vi "TAGs_AURAwheel.vi"(0 "Nº Ejes":i32[](array[numeric]), 1 "TAGs":string[](array[string]), 2 "Ejes_convoy":i32, 3 "it-LR6":i32, 4 "TAGs LR6":string[](array[string]), 5 "it-read-LR6":i32[](array[numeric]), 8 "Plataformas?":bool) -> (7 "TAGS_AURA":string[][](array[string]))   [LabVIEW 2015]
panel:
  out "x > y?":bool
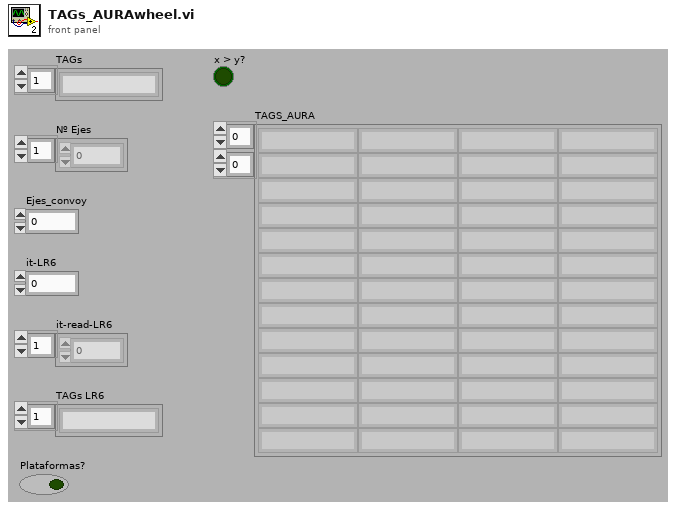
[diagram p1: front panel]
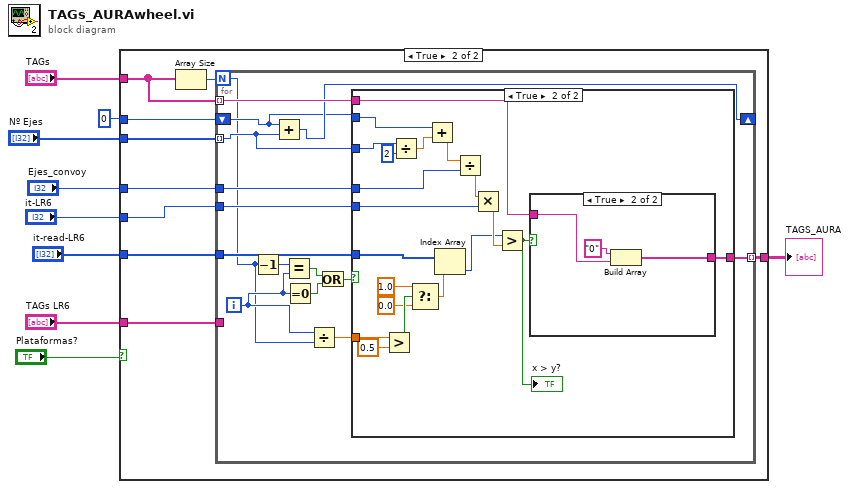
[diagram p0: block diagram]
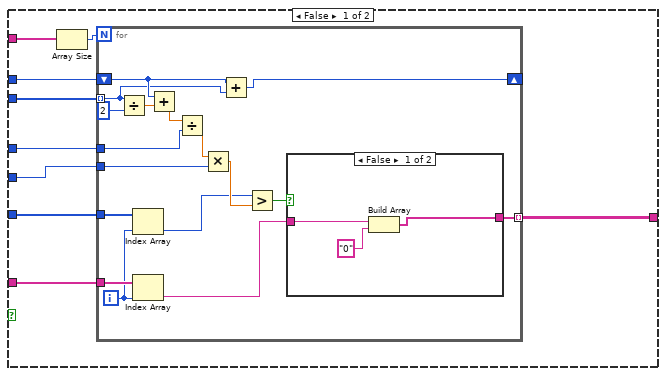
[diagram p2: hidden frame]
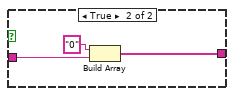
[diagram p3: hidden frame]
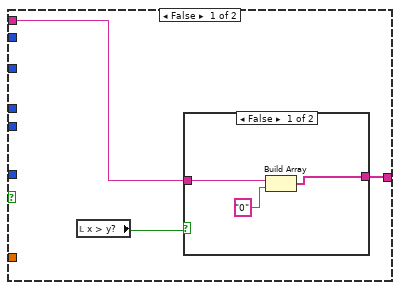
[diagram p4: hidden frame]
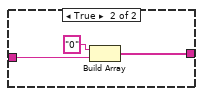
[diagram p5: hidden frame]
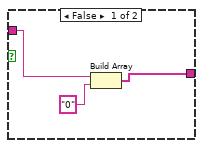
[diagram p6: hidden frame]
diagram:
  n1 = case shown="True" "Plataformas?" {
    tunnel: "TAGs LR6" -> [w17 w45]
    tunnel: "it-LR6" -> [w13 w47]
    tunnel: "it-read-LR6" -> [w16 w46]
    tunnel: "Nº Ejes" -> [w15 w49]
    tunnel: "Ejes_convoy" -> [w14 w48]
    tunnel: "TAGs" -> [w12 w43]
    tunnel: [w11 w44] -> w8
    tunnel: 0 -> [w10 w42]
    frame False {
      n2 = Array Size(array=w12) -> (size(s)=w18:i32)
      n3 = for {
        N: w18 -> [_]
        tunnel: w17 -> [w35]
        tunnel: w16 -> [w34]
        tunnel: w15 -> [w20] mode=indexing
        tunnel: w14 -> [w31]
        tunnel: w13 -> [w29]
        tunnel: [w24] -> w11 mode=indexing
        shift-right: [w19] -> _
        shift-left: w10 -> [w21]
        i -> [w33]
        n4 = Divide(x=w20, y=2) -> (x/y=w23:dbl)
        n5 = Index Array(array=w34, index=w33) -> (element=w27:i32)
        n6 = Index Array(array=w35, index=w33) -> (element=w25:string)
        n7 = Add(x=w21, y=w23) -> (x+y=w22:dbl)
        n8 = Divide(x=w22, y=w31) -> (x/y=w30:dbl)
        n9 = Multiply(x=w30, y=w29) -> (x*y=w28:dbl)
        n10 = Add(x=w21, y=w20) -> (x+y=w19:i32)
        n11 = Greater?(x=w27, y=w28) -> (0:w26:bool)
        n12 = case shown="False" w26 {
          tunnel: w25 -> [w37 w41]
          tunnel: [w36 w39] -> w24
          frame False {
            n13 = Build Array(w37, "0" ("element")) -> (w36:string[])
          }
          frame True {
            n14 = Build Array("0" ("element"), w41) -> (w39:string[])
          }
        }
      }
    }
    frame True {
      n15 = Array Size(array=w43) -> (size(s)=w50:i32)
      n16 = for {
        N: w50 -> [w52]
        tunnel: w45 -> [_]
        tunnel: w46 -> [w65]
        tunnel: w49 -> [w55] mode=indexing
        tunnel: w48 -> [w64]
        tunnel: w47 -> [w63]
        tunnel: [w62] -> w44 mode=indexing
        tunnel: w43 -> [w57] mode=indexing
        shift-right: [w56] -> _
        shift-left: w42 -> [w54]
        i -> [w53]
        n17 = Decrement(x=w52) -> (x-1=w61:i32)
        n18 = Add(x=w54, y=w55) -> (x+y=w56:i32)
        n19 = Equal?(x=w61, y=w53) -> (x = y?=w58:bool)
        n20 = Equal To 0?(x=w53) -> (x = 0?=w59:bool)
        n21 = Divide(x=w53, y=w52) -> (x/y=w51:dbl)
        n22 = Or(x=w58, y=w59) -> (x .or. y?=w60:bool)
        n23 = case shown="True" w60 {
          tunnel: w65 -> [_ w94]
          tunnel: w64 -> [_ w92]
          tunnel: w63 -> [_ w90]
          tunnel: [w67 w86] -> w62
          tunnel: w57 -> [w68 w81]
          tunnel: w55 -> [_ w85]
          tunnel: w54 -> [_ w84]
          tunnel: w51 -> [_ w80]
          frame False {
            n24 = local read "x > y?"() -> (w66:bool)
            n25 = case shown="False" w66 {
              tunnel: w68 -> [w70 w74]
              tunnel: [w69 w72] -> w67
              frame False {
                n26 = Build Array(w70, "0" ("element")) -> (w69:string[])
              }
              frame True {
                n27 = Build Array("0" ("element"), w74) -> (w72:string[])
              }
            }
          }
          frame True {
            n28 = Greater?(x=w80, y=0.5) -> (0:w78:bool)
            n29 = Divide(x=w85, y=2) -> (x/y=w83:dbl)
            n30 = Select(t=1.0, s=w78, f=0.0) -> (s? t:f=w75:dbl)
            n31 = Add(x=w84, y=w83) -> (x+y=w82:dbl)
            n32 = Index Array(array=w94, index=w75) -> (element=w88:i32)
            n33 = Divide(x=w82, y=w92) -> (x/y=w91:dbl)
            n34 = Multiply(x=w91, y=w90) -> (x*y=w89:dbl)
            n35 = Greater?(x=w88, y=w89) -> (0:w87:bool)
            "x > y?" <- w87
            n36 = case shown="True" w87 {
              tunnel: w81 -> [w96 w100]
              tunnel: [w95 w98] -> w86
              frame False {
                n37 = Build Array(w96, "0" ("element")) -> (w95:string[])
              }
              frame True {
                n38 = Build Array("0" ("element"), w100) -> (w98:string[])
              }
            }
          }
        }
      }
    }
  }
  "TAGS_AURA" <- w8
